vi "config5105.vi"(4 "error in":errorcluster, 6 "Cluster":T4 {"vertical coupling" items=["AC", "DC", "Ground"]}, 7 "instrument handle":refnum<k15>) -> (0 "error out":errorcluster, 3 "instrument handle out":refnum<k15>)   [LabVIEW 2010]
uses:
  <instrlib>/niScope/Controls/niScope vertical coupling.ctl
  <instrlib>/niScope/Controls/niScope trigger source digital.ctl
  <instrlib>/niScope/Controls/niScope trigger slope.ctl
  <instrlib>/niScope/Configure/Trigger/niScope Configure Trigger Digital.vi
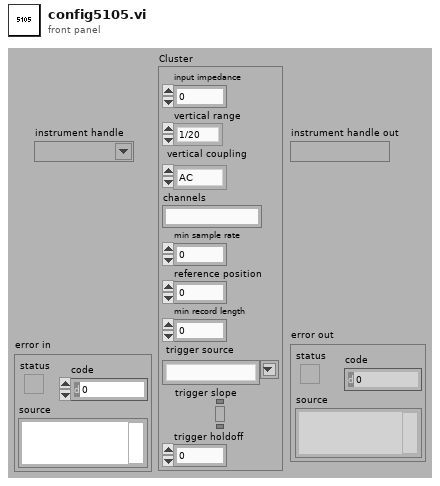
[diagram p1: front panel]
types:
  T1 = typedef "niScope vertical coupling.ctl" = i32
  T2 = typedef "niScope trigger source digital.ctl" = string
  T3 = typedef "niScope trigger slope.ctl" = i32
  T4 = cluster{"input impedance":u32, "vertical range":enum16{"1/20", "1/5", "1", "6", "30"}, "vertical coupling":T1, "channels":string, "min sample rate":dbl, "reference position":dbl, "min record length":i32, "trigger source":T2, "trigger slope":T3, "trigger holdoff":dbl}
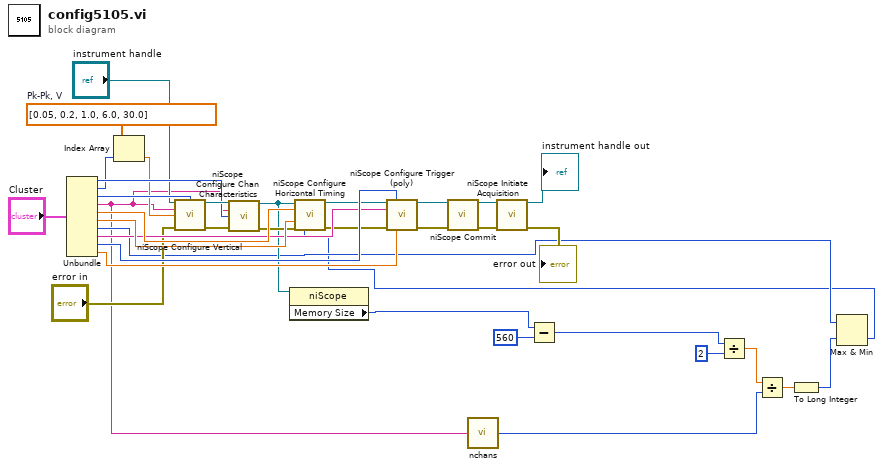
[diagram p0: block diagram]
diagram:
  w12 = dbl[] [0.05, 0.2, 1.0, 6.0, 30.0]  # Pk-Pk, V
  n1 = Unbundle("Cluster") -> ("input impedance"=w26:u32, "vertical range"=w19:enum16{"1/20", "1/5", "1", "6", "30"}, "vertical coupling"=w32:T1, "channels"=w5:string, "min sample rate"=w33:dbl, "reference position"=w34:dbl, "min record length"=w6:i32, "trigger source"=w31:T2, "trigger slope"=w35:T3, "trigger holdoff"=w36:dbl)
  n2 = Index Array(array=w12, index=w19) -> (element=w18:dbl)
  n3 = call <instrlib>:"niScope Configure Vertical.vi"("instrument handle"="instrument handle", "vertical coupling"=w32, "channels"=w5, "vertical range"=w18, "error in"="error in") -> ("instrument handle out"=w27:refnum<k15>, "error out"=w20:errorcluster)  [unwired: 9 in]
  n4 = call <instrlib>:"niScope Configure Chan Characteristics.vi"("instrument handle"=w27, "channels"=w5, "input impedance"=w26, "error in"=w20) -> ("instrument handle out"=w13:refnum<k15>, "error out"=w21:errorcluster)  [unwired: 10 in]
  n5 = property class="niScope"(reference=w13) -> ("Memory Size"=w3:i32)  [unwired: 1 in, 2 out]
  n6 = call "nchans.vi"("channels"=w5) -> ("length (rest)"=w9:i32)
  n7 = Subtract(x=w3, y=560) -> (x-y=w1:i32)
  n8 = Divide(x=w1, y=2) -> (x/y=w10:dbl)
  n9 = Divide(x=w10, y=w9) -> (x/y=w8:dbl)
  n10 = To Long Integer(number=w8) -> (32bit integer=w7:i32)
  n11 = Max & Min(x=w6, y=w7) -> (min(x,y)=w4:i32)  [unwired: 1 out]
  n12 = call <instrlib>:"niScope Configure Horizontal Timing.vi"("instrument handle"=w13, "min sample rate"=w33, "reference position"=w34, "error in"=w21, "min record length"=w4) -> ("instrument handle out"=w28:refnum<k15>, "error out"=w22:errorcluster)  [unwired: 9 in]
  n13 = call-poly <instrlib>:"niScope Configure Trigger (poly).vi"("instrument handle"=w28, "trigger slope"=w35, "trigger source"=w31, "error in"=w22, "trigger holdoff"=w36) -> ("instrument handle out"=w29:refnum<k15>, "error out"=w23:errorcluster)  [unwired: 9 in]
  n14 = call <instrlib>:"niScope Commit.vi"("instrument handle"=w29, "error in"=w23) -> ("instrument handle out"=w30:refnum<k15>, "error out"=w24:errorcluster)  [unwired: 12 in]
  n15 = call <instrlib>:"niScope Initiate Acquisition.vi"("instrument handle"=w30, "error in"=w24) -> ("instrument handle out"=→"instrument handle out":refnum<k15>, "error out"=→"error out":errorcluster)  [unwired: 12 in]
